vi "Absolute Difference.vi"() -> ()   [LabVIEW 2014]
doc: "Use this template to build a VI to use as a subVI."
uses:
  <vilib>/vision/NI_Vision_Development_Module.lvlib
panel:
  out "Src":T1(plugin-control)
  out "Dst":T1(plugin-control)
  # ":: MVi Framework V1.0 ::\nAuthor:Gaoke Yang\nEmail: gaoke.yang@yahoo.com\nWeb: www.mvicontrol.com\nCopyright (C) 2015, MVI Technologies All Rights Reserved"
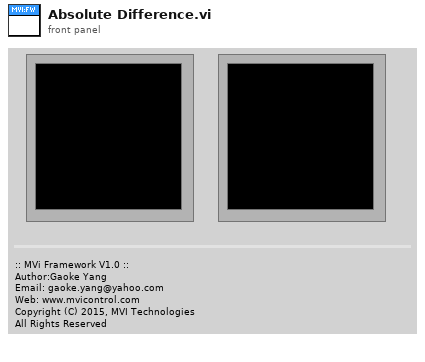
[diagram p1: front panel]
types:
  T1 = typedef "IMAQ Image.ctl" = refnum<image>
  T2 = cluster{"X Size":i32, "Y Size":i32, "% Tolerance":i32}
  T3 = typedef "Image Type" = u32
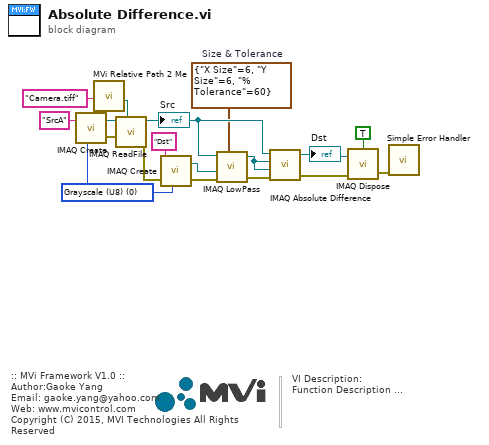
[diagram p0: block diagram]
diagram:
  w2 = T2 {"X Size"=6, "Y Size"=6, "% Tolerance"=60}  # Size & Tolerance
  w11 = T3 0 items=["Grayscale (U8)", "Grayscale (I16)", "Grayscale (SGL)", "Complex (CSG)", "RGB (U32)", "HSL (U32)", "RGB (U64)", "Grayscale (U16)"] ("Image Type")
  # "VI Description:\nFunction Description ..."
  # ":: MVi Framework V1.0 ::\nAuthor:Gaoke Yang\nEmail: gaoke.yang@yahoo.com\nWeb: www.mvicontrol.com\nCopyright (C) 2015, MVI Technologies All Rights Reserved"
  n1 = call "IMAQ Create"("Image Name"="SrcA" ("name or relative path"), "Image Type"=w11) -> ("New Image"=w12:T1, "error out"=w10:errorcluster)  [unwired: 2 in, 1 out]
  n2 = call "MVi Relative Path 2 Me.vi"("Relative Path"="Camera.tiff" ("name or relative path")) -> ("Appended Dir"=w14:path)  [unwired: 5 in, 1 out]
  n3 = call "IMAQ ReadFile"("File Path"=w14, "error in (no error)"=w10, "Image"=w12) -> ("error out"=w1:errorcluster, "Image Out"=w8:T1)  [unwired: 4 in, 3 out]
  "Src" <- w8
  n4 = call "IMAQ Create"("Image Name"="Dst" ("name or relative path"), "Image Type"=w11, "error in (no error)"=w1) -> ("New Image"=w6:T1, "error out"=w7:errorcluster)  [unwired: 1 in, 1 out]
  n5 = call "IMAQ LowPass"("Image Src"=w8, "Size & Tolerance"=w2, "Image Dst"=w6, "error in (no error)"=w7) -> ("Image Dst Out"=w5:T1, "error out"=w3:errorcluster)  [unwired: 3 in]
  n6 = call "IMAQ Absolute Difference"("Image Src A"=w8, "Image Dst"=w5, "Image Src B"=w5, "error in (no error)"=w3) -> ("Image Dst Out"=w9:T1, "error out"=w4:errorcluster)  [unwired: 3 in]
  "Dst" <- w9
  n7 = call "IMAQ Dispose"("All Images? (No)"=TRUE, "Image"=w9, "error in (no error)"=w4) -> ("error out"=w15:errorcluster)  [unwired: 3 out]
  n8 = call <vilib>:"Simple Error Handler.vi"("error in (no error)"=w15) -> ()  [unwired: 1 in, 8 out]
